vi "Read Filename.vi"(8 "error in (no error)":errorcluster, 11 "CFitsIO in":refnum<class "CFitsIO.lvclass">) -> (0 "error out":errorcluster, 2 "Filename":string, 3 "CFitsIO out":refnum<class "CFitsIO.lvclass">)   [LabVIEW 2016, in "CFitsIO.lvclass"]
uses:
  CFitsIO.lvclass
  CFitsIO.lvclass/CFitsIO.ctl
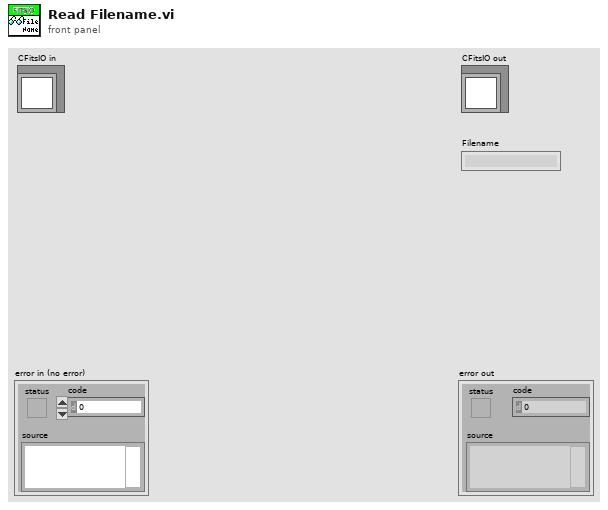
[diagram p1: front panel]
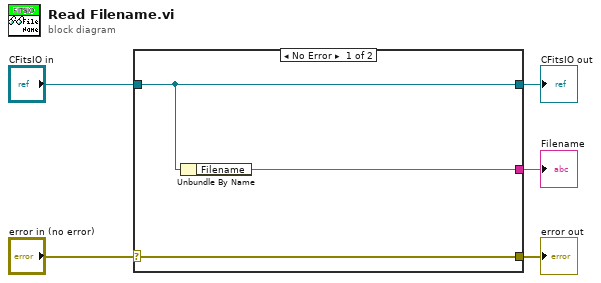
[diagram p0: block diagram]
diagram:
  n1 = case shown="No Error" "error in (no error)" {
    selector: "error in (no error)" -> [w8 w9]
    tunnel: [w8 w9] -> w4
    tunnel: [w7 w10] -> w2
    tunnel: "CFitsIO in" -> [w7 w10]
    tunnel: [w6 _] -> w1
    frame No Error {
      n2 = Unbundle By Name(w7) -> ("Filename"=w6:string)
    }
    frame Error {
    }
  }
  "error out" <- w4
  "CFitsIO out" <- w2
  "Filename" <- w1
